vi "encoderposition(SubVI).vi"(11 "Encoder Position":dbl) -> (2 "Sine":i32(graph), 3 "Counter Value":i32)   [LabVIEW 2017]
uses:
  <vilib>/addons/control/pid/pid.llb/PID (DBL).vi
  <vilib>/addons/control/pid/NI_PID_pid.lvlib
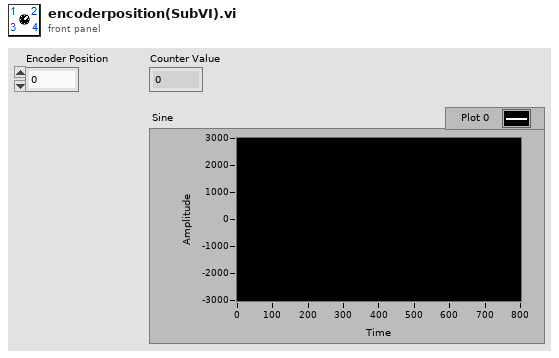
[diagram p1: front panel]
types:
  T1 = cluster{"proportional gain (Kc)":dbl, "integral time (Ti, min)":dbl, "derivative time (Td, min)":dbl}
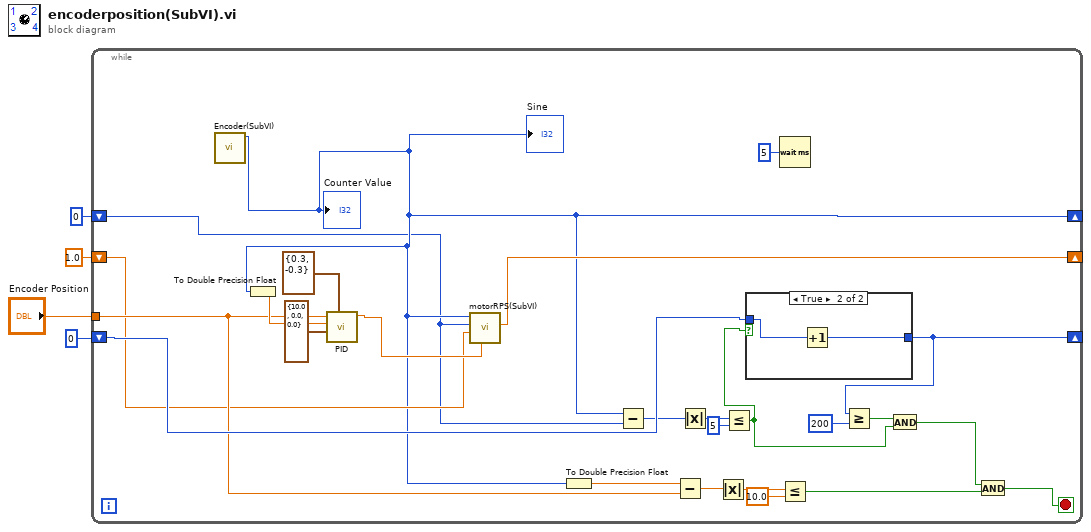
[diagram p0: block diagram]
diagram:
  n1 = while {
    tunnel: "Encoder Position" -> [w19]
    shift-right: [w10] -> _
    shift-left: 0 ("Counter Value") -> [w9]
    shift-right: [w24] -> _
    shift-left: 0 -> [w25]
    shift-right: [w12] -> _
    shift-left: 1.0 ("dt out (s) out") -> [w11]
    stop <- w20 stop-if-true
    n2 = call "Encoder(SubVI).vi"() -> ("Counter Value"=w10:i32)  [unwired: 10 in, 1 out]
    "Sine" <- w10
    "Counter Value" <- w10
    n3 = To Double Precision Float(number=w10) -> (double precision float=w29:dbl)
    n4 = call-poly <vilib>:"PID.vi"("output range"=cluster{"output high":dbl, "output low":dbl} {"output high"=0.3, "output low"=-0.3}, "PID gains"=T1 {"proportional gain (Kc)"=10.0, "integral time (Ti, min)"=0.0, "derivative time (Td, min)"=0.0}, "process variable"=w29, "setpoint"=w19) -> ("output"=w13:dbl)  [unwired: 6 in, 1 out]
    n5 = call "motorRPS(SubVI).vi"("desired rps"=w13, "dt out (s) in"=w11, "Previous Encoder Value"=w9, "Current Encoder Value"=w10) -> ("dt out (s) out"=w12:dbl)  [unwired: 5 in, 2 out]
    n6 = To Double Precision Float(number=w10) -> (double precision float=w18:dbl)
    n7 = Subtract(x=w10, y=w9) -> (x-y=w8:i32)
    n8 = Subtract(x=w18, y=w19) -> (x-y=w17:dbl)
    n9 = Absolute Value(x=w8) -> (abs(x)=w7:i32)
    n10 = Absolute Value(x=w17) -> (abs(x)=w16:dbl)
    n11 = Less Or Equal?(x=w7, y=5) -> (x <= y?=w5:bool)
    n12 = case shown="True" w5 {
      tunnel: w25 -> [w30 w32]
      tunnel: [w30 w31] -> w24
      frame False {
      }
      frame True {
        n13 = Increment(x=w32) -> (x+1=w31:i32)
      }
    }
    n14 = Wait (ms)(milliseconds to wait=u32 5) -> ()  [unwired: 1 out]
    n15 = Less Or Equal?(x=w16, y=10.0) -> (x <= y?=w14:bool)
    n16 = Greater Or Equal?(x=w24, y=200) -> (x >= y?=w22:bool)
    n17 = And(x=w22, y=w5) -> (x .and. y?=w21:bool)
    n18 = And(x=w21, y=w14) -> (x .and. y?=w20:bool)
  }
